vi "PV ActiveLine - Test IO.vi"(7 "W/R":bool, 8 "Fehler (Eingang)":errorcluster, 9 "Relay status":u8(ring) items=[" All relays deactivated", " Switching function relay 1 activated", " Switching function relay 2 activated", " Switching function relay 3 activated", " Switching function relay 4 activated", "Gauge relay CH1 activated", "Gauge relay activated", "Error relay activated", "All relays activated"], 10 "I / O Test":u8(ring) items=[" Test stopped", " Test runs"], 11 "Referenz in":refnum<visa-resource-name>) -> (0 "Cluster (Ausgang)":errorcluster, 1 "Relay status out":string, 2 "Get I / O Test":u8(ring) items=[" Test stopped", " Test runs"], 3 "Referenz out":refnum<visa-resource-name>)   [LabVIEW 2013, in "PV ActiveLine.lvlib"]
doc: "TIO I/O Test --> TIO replaced the IOT (old) command\n\nTest status,\na =\n0 –> Test stopped\n1 –> Test runs\n\nRelay status (in hex format),\nbb =\n00 –> All relays deactivated\n01 –> Switching function relay 1 activated\n02 –> Switching function relay 2 activated\n04 –> Switching function relay 3 activated\n08 –> Switching function relay 4 activated\n40 –> Error relay activated\n4F –> All relays activated\n\nCaution: \nThe relays switch irrespective of the pressure. \nStarting a test program may cause unwanted effects in connected control systems.\nDisconnect all sensor cables and control system lines to ensure that no control commands or messages are triggered by mistake."
uses:
  <instrlib>/PV ActiveLine/PV ActiveLine.lvlib
panel:
  # "Caution\nCaution: The relays switch irrespective of the pressure.\nStarting a test program may cause unwanted effects in connected\ncontrol systems.\nDisconnect all sensor cables and control system lines to ensure that\nno control commands or messages are triggered by mistake."
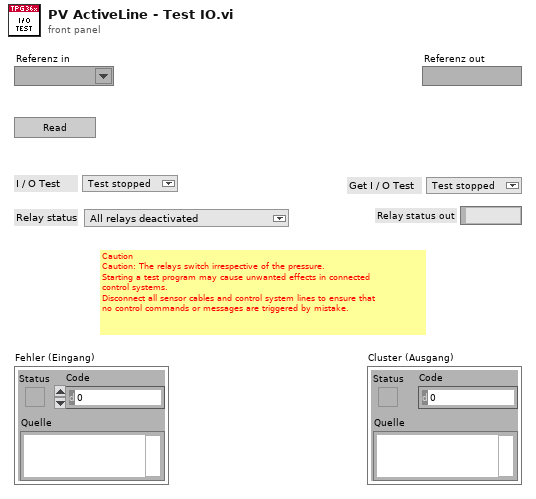
[diagram p1: front panel]
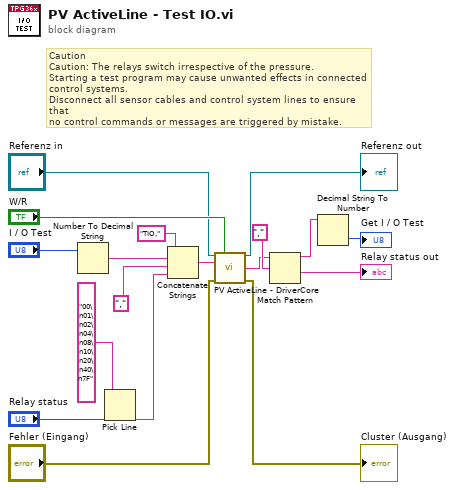
[diagram p0: block diagram]
diagram:
  # "Caution\nCaution: The relays switch irrespective of the pressure.\nStarting a test program may cause unwanted effects in connected\ncontrol systems.\nDisconnect all sensor cables and control system lines to ensure that\nno control commands or messages are triggered by mistake."
  n1 = Number To Decimal String(number="I / O Test") -> (decimal integer string=w13:string)  [unwired: 1 in]
  n2 = Pick Line(multi-line string="00\n01\n02\n04\n08\n10\n20\n40\n7F" ("Command"), line index="Relay status") -> (output string=w9:string)  [unwired: 1 in]
  n3 = Concatenate Strings("TIO," ("Command"), w13, "," ("Command"), w9) -> (w5:string)
  n4 = call <instrlib>:"PV ActiveLine - DriverCore.vi"("Referenz in"="Referenz in", "Write/Read"="W/R", "Command"=w5, "Fehler (Eingang)"="Fehler (Eingang)") -> ("Referenz out"=→"Referenz out":refnum<visa-resource-name>, "String Out"=w7:string, "Cluster (Ausgang)"=→"Cluster (Ausgang)":errorcluster)  [unwired: 9 in]
  n5 = Match Pattern(string=w7, regular expression=",") -> (before substring=w6:string, after substring=→"Relay status out":string)  [unwired: 1 in, 2 out]
  n6 = Decimal String To Number(string=w6) -> (number=→"Get I / O Test":i32)  [unwired: 2 in, 1 out]
